vi "Write IGObjectFactory.vi"(10 "IGObjectFactory":refnum<class "IGObjectFactory.lvclass">, 11 "Project in":refnum<class "Project.lvclass">) -> (3 "Project out":refnum<class "Project.lvclass">)   [LabVIEW 2016, in "Project.lvclass"]
uses:
  Project.lvclass
  IGObjectFactory/IGObjectFactory.lvclass
  Project.lvclass/Project.ctl
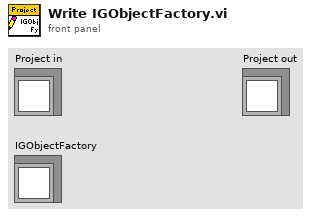
[diagram p1: front panel]
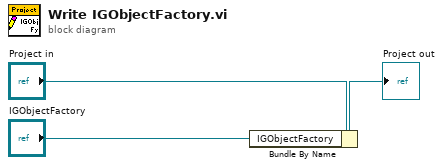
[diagram p0: block diagram]
diagram:
  n1 = Bundle By Name(cluster="Project in", "IGObjectFactory"="IGObjectFactory") -> (→"Project out":refnum<class "Project.lvclass">)
